vi "CreateLogRolloverNode.vi"(7 "DOM Document":refnum<k20>, 8 "Error In":errorcluster, 11 "Log Rollover Configuration":T1) -> (0 "Error Out":errorcluster, 3 "Rollover Node":refnum<k20>)   [LabVIEW 2012]
uses:
  LogRolloverConfiguration.ctl
  LogRolloverTriggerType.ctl
  LogDigitalIOTriggerEdge.ctl
  libs/LV-Utilities/LV-Utilities.lvlib
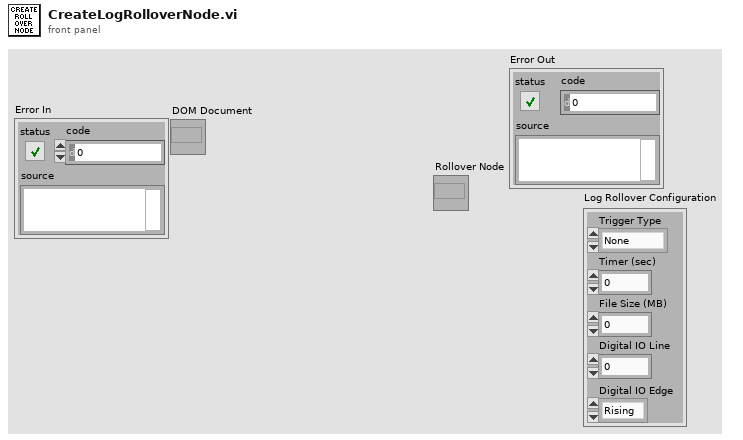
[diagram p1: front panel]
types:
  T1 = typedef "LogRolloverConfiguration.ctl" = cluster{"Trigger Type":T2, "Timer (sec)":dbl, "File Size (MB)":u32, "Digital IO Line":u8, "Digital IO Edge":T3}
  T2 = typedef "LogRolloverTriggerType.ctl" = enum16{"None", "Timer", "File Size", "Digital IO"}
  T3 = typedef "LogDigitalIOTriggerEdge.ctl" = enum16{"Rising", "Falling"}
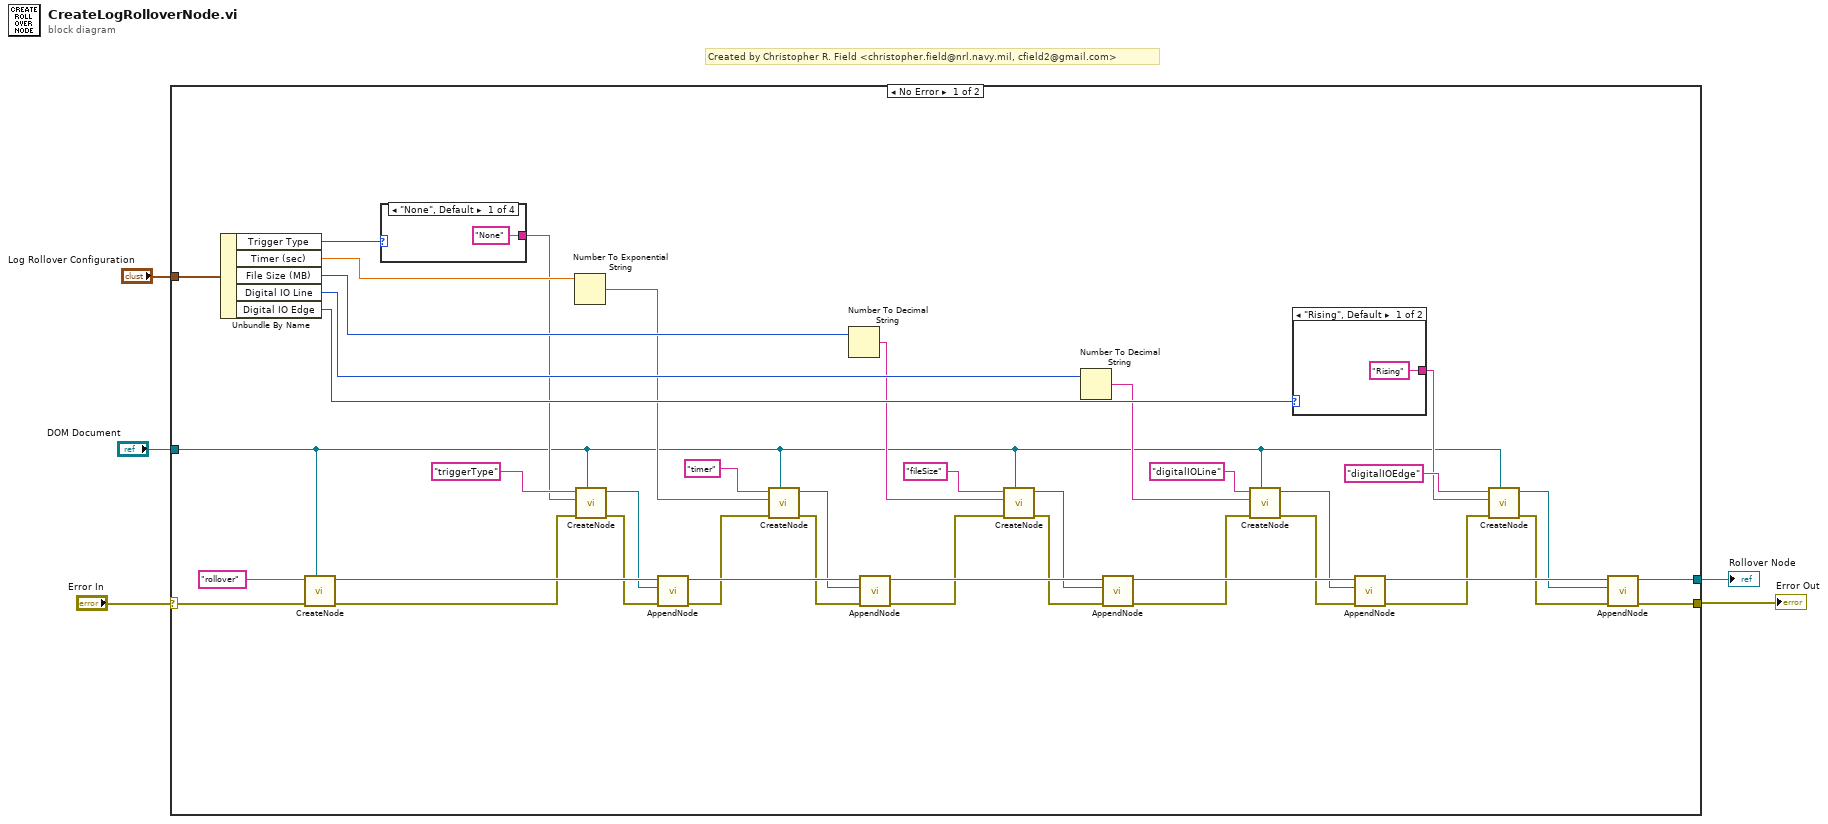
[diagram p0: block diagram]
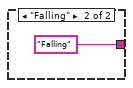
[diagram p2: hidden frame]
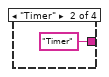
[diagram p3: hidden frame]
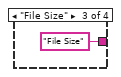
[diagram p4: hidden frame]
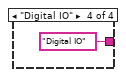
[diagram p5: hidden frame]
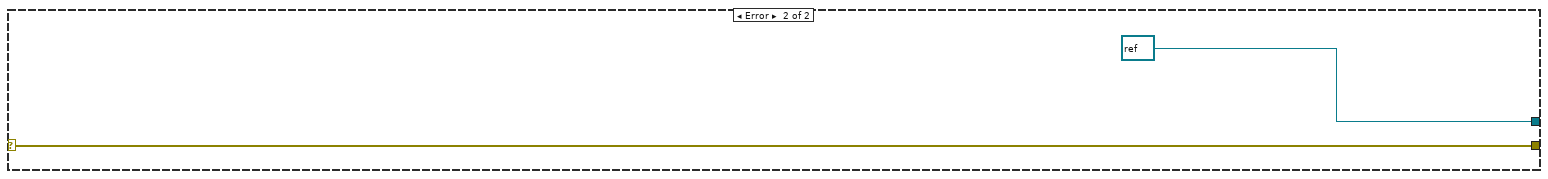
[diagram p6: hidden frame]
diagram:
  # "Created by Christopher R. Field <christopher.field@nrl.navy.mil, cfield2@gmail.com>"
  n1 = case shown="No Error" "Error In" {
    selector: "Error In" -> [w29 w54]
    tunnel: "DOM Document" -> [w24 _]
    tunnel: [w19 refnum<k20> refnum ("Wirings Node 2")] -> w3
    tunnel: [w18 w54] -> w2
    tunnel: "Log Rollover Configuration" -> [w46 _]
    frame No Error {
      n2 = Unbundle By Name(w46) -> ("Trigger Type"=w45:T2, "Timer (sec)"=w44:dbl, "File Size (MB)"=w43:u32, "Digital IO Line"=w41:u8, "Digital IO Edge"=w42:T3)
      n3 = call "CreateNode.vi"("DOM Document"=w24, "Error In"=w29, "Tag Name"="rollover") -> ("Error out"=w25:errorcluster, "Node"=w28:refnum<k20>)  [unwired: 7 in]
      n4 = case shown="\"None\", Default" w45 {
        tunnel: ["None" "Timer" "File Size" "Digital IO"] -> w31
        frame "None", Default {
        }
        frame "Timer" {
        }
        frame "File Size" {
        }
        frame "Digital IO" {
        }
      }
      n5 = Number To Exponential String(number=w44) -> (E-format string=w32:string)  [unwired: 3 in]
      n6 = call "CreateNode.vi"("DOM Document"=w24, "Error In"=w25, "Text"=w31, "Tag Name"="triggerType") -> ("Error out"=w26:errorcluster, "Node"=w27:refnum<k20>)  [unwired: 6 in]
      n7 = call "AppendNode.vi"("Error In"=w26, "Child Node"=w27, "Parent Node In"=w28) -> ("Error Out"=w6:errorcluster, "Parent Node Out"=w23:refnum<k20>)  [unwired: 7 in]
      n8 = call "CreateNode.vi"("DOM Document"=w24, "Error In"=w6, "Text"=w32, "Tag Name"="timer") -> ("Error out"=w8:errorcluster, "Node"=w7:refnum<k20>)  [unwired: 6 in]
      n9 = Number To Decimal String(number=w43) -> (decimal integer string=w33:string)  [unwired: 1 in]
      n10 = call "AppendNode.vi"("Error In"=w8, "Child Node"=w7, "Parent Node In"=w23) -> ("Error Out"=w9:errorcluster, "Parent Node Out"=w22:refnum<k20>)  [unwired: 7 in]
      n11 = call "CreateNode.vi"("DOM Document"=w24, "Error In"=w9, "Text"=w33, "Tag Name"="fileSize" ("Text")) -> ("Error out"=w11:errorcluster, "Node"=w10:refnum<k20>)  [unwired: 6 in]
      n12 = Number To Decimal String(number=w41) -> (decimal integer string=w34:string)  [unwired: 1 in]
      n13 = call "AppendNode.vi"("Error In"=w11, "Child Node"=w10, "Parent Node In"=w22) -> ("Error Out"=w12:errorcluster, "Parent Node Out"=w21:refnum<k20>)  [unwired: 7 in]
      n14 = call "CreateNode.vi"("DOM Document"=w24, "Error In"=w12, "Text"=w34, "Tag Name"="digitalIOLine") -> ("Error out"=w13:errorcluster, "Node"=w14:refnum<k20>)  [unwired: 6 in]
      n15 = case shown="\"Rising\", Default" w42 {
        tunnel: ["Rising" "Falling"] -> w35
        frame "Rising", Default {
        }
        frame "Falling" {
        }
      }
      n16 = call "AppendNode.vi"("Error In"=w13, "Child Node"=w14, "Parent Node In"=w21) -> ("Error Out"=w15:errorcluster, "Parent Node Out"=w20:refnum<k20>)  [unwired: 7 in]
      n17 = call "CreateNode.vi"("DOM Document"=w24, "Error In"=w15, "Text"=w35, "Tag Name"="digitalIOEdge") -> ("Error out"=w17:errorcluster, "Node"=w16:refnum<k20>)  [unwired: 6 in]
      n18 = call "AppendNode.vi"("Error In"=w17, "Child Node"=w16, "Parent Node In"=w20) -> ("Error Out"=w18:errorcluster, "Parent Node Out"=w19:refnum<k20>)  [unwired: 7 in]
    }
    frame Error {
    }
  }
  "Rollover Node" <- w3
  "Error Out" <- w2
